vi "Dequeue Message.vi"(8 "에러 입력(에러 없음)":errorcluster, 11 "큐 입력":refnum<queue>) -> (0 "에러 출력":errorcluster, 1 "값":variant, 2 "메세지":string, 3 "큐 출력":refnum<queue>)   [LabVIEW 2020]
uses:
  Controls/Message Cluster.ctl
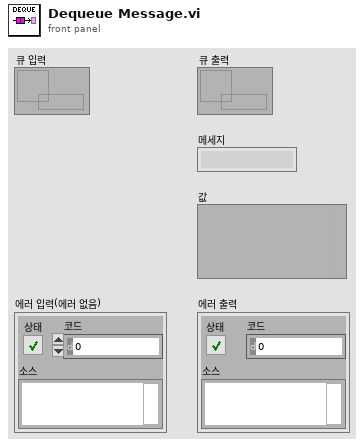
[diagram p1: front panel]
types:
  T1 = typedef "Message Cluster.ctl" = cluster{"메세지":string, "값":variant}
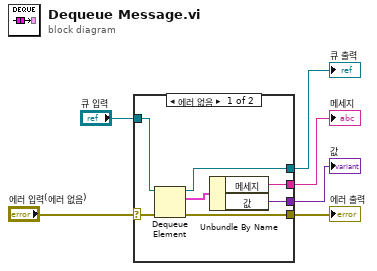
[diagram p0: block diagram]
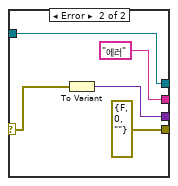
[diagram p2: hidden frame]
diagram:
  n1 = case shown="에러 없음" "에러 입력(에러 없음)" {
    selector: "에러 입력(에러 없음)" -> [w10 w15]
    tunnel: [w13 w17] -> w6
    tunnel: [w12 errorcluster {"status"=FALSE, "code"=0, "source"=""} ("error out")] -> w5
    tunnel: "큐 입력" -> [w11 w17]
    tunnel: [w8 "에러" ("메세지")] -> w2
    tunnel: [w7 w14] -> w1
    frame No Error {
      n2 = Dequeue Element(queue=w11, error in (no error)=w10) -> (queue out=w13:refnum<queue>, element=w9:T1, error out=w12:errorcluster)  [unwired: 1 in, 1 out]
      n3 = Unbundle By Name(w9) -> ("메세지"=w8:string, "값"=w7:variant)
    }
    frame Error {
      n4 = To Variant(anything=w15) -> (Variant=w14:variant)
    }
  }
  "큐 출력" <- w6
  "에러 출력" <- w5
  "값" <- w1
  "메세지" <- w2
